vi "Set Xtal Freq.vi"(8 "error in (no error)":errorcluster, 9 "Tuner Frequency":u32, 10 "RTL Frequency":u32, 11 "RTL-SDR in":refnum<class "RTL-SDR.lvclass">) -> (0 "error out":errorcluster, 1 "function return":i32, 3 "RTL-SDR out":refnum<class "RTL-SDR.lvclass">)   [LabVIEW 2015, in "RTL-SDR.lvclass"]
uses:
  RTL-SDR.lvclass
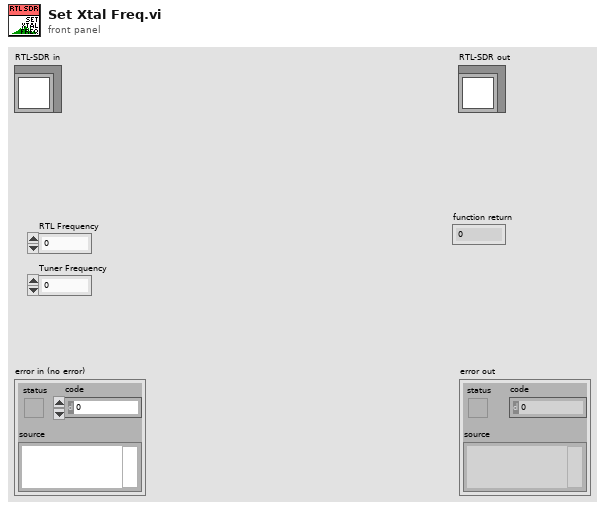
[diagram p1: front panel]
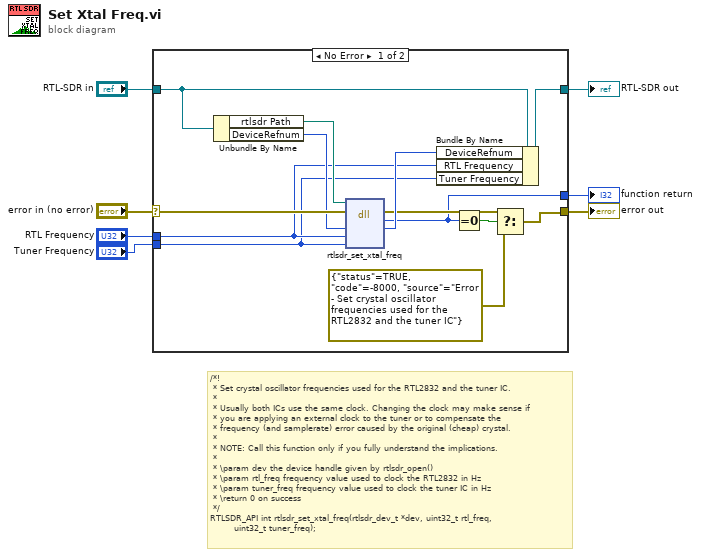
[diagram p0: block diagram]
diagram:
  # "/*!\n * Set crystal oscillator frequencies used for the RTL2832 and the tuner IC.\n *\n * Usually both ICs use the same clock. Changing the clock may make sense if\n * you are applying an external clock to the tuner or to compensate the\n * frequency (and samplerate) error caused by the original (cheap) crystal.\n *\n * NOTE: Call this function only if you fully understand the implications.\n *\n * \\param dev the device handle given by rtlsdr_open()\n * \\param rtl_freq frequency value used to clock the RTL2832 in Hz\n * \\param tuner_freq frequency value used to clock the tuner IC in Hz\n * \\return 0 on success\n */\nRTLSDR_API int rtlsdr_set_xtal_freq(rtlsdr_dev_t *dev, uint32_t rtl_freq,\n\t\t\t\t    uint32_t tuner_freq);"
  n1 = case shown="No Error" "error in (no error)" {
    selector: "error in (no error)" -> [w20 w22]
    tunnel: [w9 w22] -> w6
    tunnel: [w18 w21] -> w4
    tunnel: "RTL-SDR in" -> [w19 w21]
    tunnel: [w8 _] -> w3
    tunnel: "RTL Frequency" -> [w14 _]
    tunnel: "Tuner Frequency" -> [w13 _]
    frame No Error {
      n2 = Unbundle By Name(w19) -> ("rtlsdr Path"=w17:path, "DeviceRefnum"=w16:u64)
      n3 = dll-call lib="C:/Program Files (x86)/National Instruments/LabVIEW 2016/user.lib/rtlsdr/rtlsdr.*" fn="rtlsdr_set_xtal_freq"(path in=w17, error in=w20, "DeviceRefnum"=w16, "RTL Frequency"=w14, "Tuner Frequency"=w13) -> (error out=w10:errorcluster, "return type"=w8:i32, "DeviceRefnum"=w15:u64)  [unwired: 3 in, 1 out]
      n4 = Bundle By Name(cluster=w19, "DeviceRefnum"=w15, "RTL Frequency"=w14, "Tuner Frequency"=w13) -> (w18:refnum<class "RTL-SDR.lvclass">)
      n5 = Equal To 0?(x=w8) -> (x = 0?=w11:bool)
      n6 = Select(t=w10, s=w11, f=errorcluster {"status"=TRUE, "code"=-8000, "source"="Error - Set crystal oscillator frequencies used for the RTL2832 and the tuner IC"} ("error out")) -> (s? t:f=w9:errorcluster)
    }
    frame Error {
    }
  }
  "error out" <- w6
  "RTL-SDR out" <- w4
  "function return" <- w3
